vi "Get 1D Array String.vi"(5 "use temporary file? (F)":bool, 7 "data type of variable":string[](array[string]), 8 "error in":errorcluster, 10 "variable name":string, 11 "GOLPI ref. in":T1={"pipe handle"={"lv_proc.dll file path"=path "", "process instance handle"=[], "debug mode"=FALSE, "debug data"=[]}, "fast read timeout [ms]"=500, "fast read settle time [ms]"=10, "fast read to multiple [ms]"=1, "max elements per input line"=100, "slow read timeout [ms]"=5000, "stdin double format specifier"="%_16e", "max elements per stdout output column"=100, "console mode bitstream"=FALSE, "bitstream first read timeout [ms]"=1000, "bitstream read timeout [ms]"=50, "struct transfer possible"=FALSE, "matlab mode"=FALSE}) -> (0 "error out":errorcluster, 2 "value":string[](array[string]), 3 "GOLPI ref. out":T1={"pipe handle"={"lv_proc.dll file path"=path "", "process instance handle"=[], "debug mode"=FALSE, "debug data"=[]}, "fast read timeout [ms]"=500, "fast read settle time [ms]"=10, "fast read to multiple [ms]"=1, "max elements per input line"=100, "slow read timeout [ms]"=5000, "stdin double format specifier"="%_16e", "max elements per stdout output column"=100, "console mode bitstream"=FALSE, "bitstream first read timeout [ms]"=1000, "bitstream read timeout [ms]"=50, "struct transfer possible"=FALSE, "matlab mode"=FALSE})   [LabVIEW 2020, in "GOLPI library.lvlib"]
doc: "Part of polymorph Get Variable.vi"
uses:
  GOLPI library.lvlib
  GOLPI reference Type Def.ctl
  Pipe Handle.ctl
  Bitstream Data Type.ctl
  Custom Error Codes Enum Type Def.vi
  LV Process library.lvlib
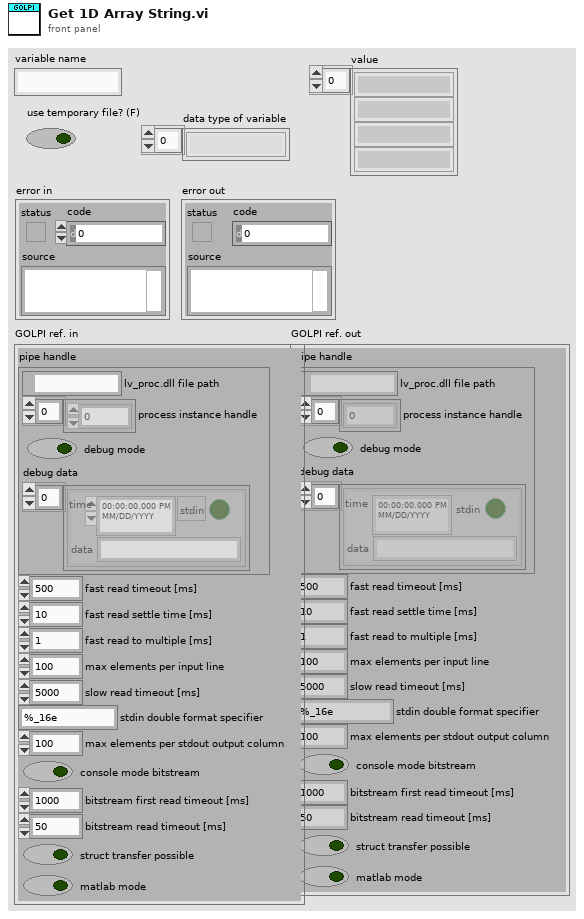
[diagram p1: front panel]
types:
  T1 = typedef "GOLPI library.lvlib/GOLPI reference Type Def.ctl" = cluster{"pipe handle":T2, "fast read timeout [ms]":u32, "fast read settle time [ms]":u32, "fast read to multiple [ms]":u32, "max elements per input line":u32, "slow read timeout [ms]":u32, "stdin double format specifier":string, "max elements per stdout output column":u32, "console mode bitstream":bool, "bitstream first read timeout [ms]":u32, "bitstream read timeout [ms]":u32, "struct transfer possible":bool, "matlab mode":bool}
  T2 = typedef "LV Process library.lvlib/Pipe Handle.ctl" = cluster{"lv_proc.dll file path":path, "process instance handle":u32[], "debug mode":bool, "debug data":cluster{"time":timestamp, "stdin":bool, "data":string}[]}
  T3 = typedef "GOLPI library.lvlib/Bitstream Data Type.ctl" = enum16{"dummy", "int", "uint", "float", "complex", "str", "real numeric"}
  T4 = typedef "GOLPI library.lvlib/Custom Error Codes Enum Type Def.vi" = enum16{"no error", "00 working directory PAR1 missing", "01 octave binary PAR1 missing", "02 octave report error PAR1", "03 empty output last cmd PAR1", "04 missing temporary file PAR1", "05 pwd PAR 1 not exist", "06 oct package not installed", "07 octave default binary missing", "10 var PAR1 not string, vect", "11 var PAR1 not num, scal, ~compl", "12 var PAR1 not num, scal, compl", "13 var PAR1 not num, vect, ~compl", "14 var PAR1 not num, vect, compl", "15 var PAR1 not num, mat, ~compl", "16 var PAR1 not num, mat, ~compl", "30 read timeout", "60 bitstream transport failed", "61 bitstream decode error PAR1", "62 bitstream cannot be set", "70 struct transfer not possible", "80 struct: cluster elem. PAR1 not implem.", "81 struct: structure field PAR1 not implem.", "82 struct: size mismatch of PAR1", "83 struct: type mismatch of PAR1", "98 internal error", "99 not finished", "90 Not supported in Matlab mode", "91 Matlab variable transfer error", "92 Matlab Script Error"}
  T5 = typedef "GOLPI library.lvlib/Bitstream Data.ctl" = cluster{"double":dbl[][], "cplx double":cdb[][], "int64":i64[][], "uint64":u64[][], "str":string[], "data type":T3}
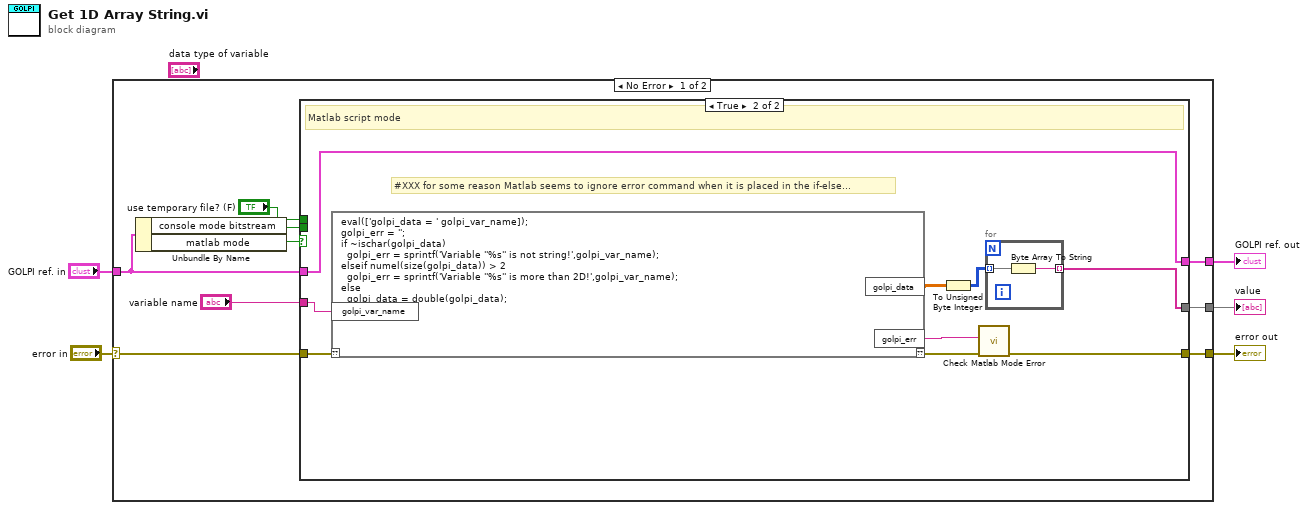
[diagram p0: block diagram]
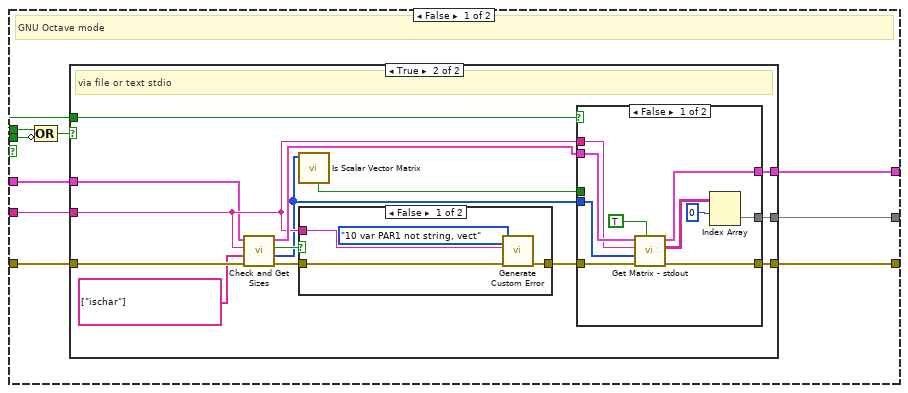
[diagram p2: hidden frame]
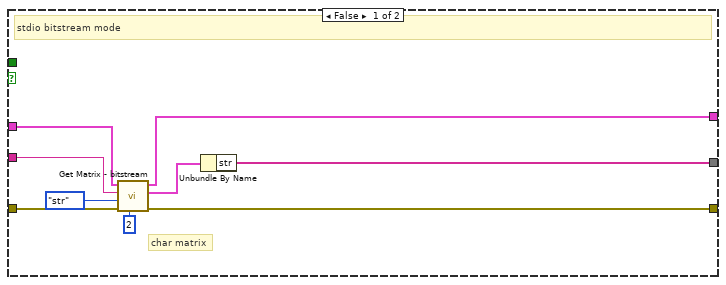
[diagram p3: hidden frame]
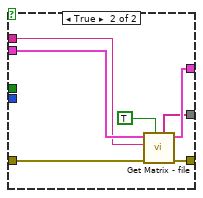
[diagram p4: hidden frame]
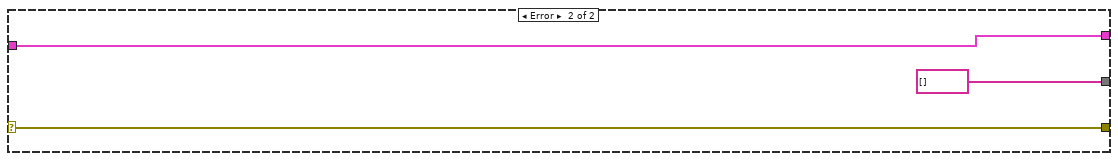
[diagram p6: hidden frame]
diagram:
  n1 = case shown="No Error" "error in" {
    selector: "error in" -> [w13 w82]
    tunnel: [w12 w82] -> w5
    tunnel: [w14 string[] [] ("vector")] -> w3
    tunnel: "GOLPI ref. in" -> [w9 w80]
    tunnel: [w10 w80] -> w1
    frame No Error {
      n2 = Unbundle By Name(w9) -> ("console mode bitstream"=w8:bool, "matlab mode"=w6:bool)
      n3 = case shown="True" w6 {
        tunnel: [w23 w72] -> w14
        tunnel: w13 -> [w22 w77]
        tunnel: [w21 w69] -> w12
        tunnel: "variable name" -> [w20 w76]
        tunnel: [w19 w75] -> w10
        tunnel: w9 -> [w18 w75]
        tunnel: w8 -> [w17 _]
        tunnel: "use temporary file? (F)" -> [w15 _]
        frame False {
          # "GNU Octave mode"
          n4 = Compound Arithmetic op=OR(w15, invert w17) -> (w16:bool)
          n5 = case shown="True" w16 {
            tunnel: [w25 w46] -> w23
            tunnel: w22 -> [w32 w44]
            tunnel: [w24 w39] -> w21
            tunnel: w20 -> [w29 w38]
            tunnel: w18 -> [w31 w37]
            tunnel: [w30 w36] -> w19
            tunnel: w15 -> [_ w33]
            frame False {
              # "char matrix"
              # "stdio bitstream mode"
              n6 = call "Get Matrix - bitstream.vi"("max dimensions (0: scalar)"=2, "error in (no error)"=w32, "data type"=Bitstream_Data_Type."str", "variable name"=w29, "GOLPI ref. in"=w31) -> ("error out"=w24:errorcluster, "data"=w26:T5, "GOLPI ref. out"=w30:T1)  [unwired: 4 in]
              n7 = Unbundle By Name(w26) -> ("str"=w25:string[])
            }
            frame True {
              # "via file or text stdio"
              n8 = call "Check and Get Sizes.vi"("error in (no error)"=w44, "test commands"=string[] ["ischar"], "variable name"=w38, "GOLPI ref. in"=w37) -> ("error out"=w43:errorcluster, "octave sizes"=w35:i32[], "all tests OK?"=w45:bool, "GOLPI ref. out"=w41:T1)  [unwired: 4 in]
              n9 = call "Is Scalar Vector Matrix.vi"("octave sizes"=w35) -> ("row vector?"=w34:bool)  [unwired: 5 in, 5 out]
              n10 = case shown="False" w45 {
                tunnel: w43 -> [w67 w68]
                tunnel: [w64 w68] -> w40
                tunnel: w38 -> [w65 _]
                frame False {
                  n11 = call "Generate Custom Error.vi"("error in"=w67, "PAR1"=w65, "GOLPI error"=Custom_Error_Codes_Enum_Type_Def.vi."10 var PAR1 not string, vect" ("Enum")) -> ("error out"=w64:errorcluster)  [unwired: 8 in]
                }
                frame True {
                }
              }
              n12 = case shown="False" w33 {
                tunnel: [w47 w58] -> w46
                tunnel: w41 -> [w56 w61]
                tunnel: w35 -> [w49 _]
                tunnel: w40 -> [w55 w63]
                tunnel: [w54 w62] -> w39
                tunnel: w38 -> [w48 w59]
                tunnel: [w53 w60] -> w36
                tunnel: w34 -> [_ _]
                frame False {
                  n13 = call "Get Matrix - stdout.vi"("is string?"=TRUE ("is string"), "error in (no error)"=w55, "octave sizes"=w49, "variable name"=w48, "GOLPI ref. in"=w56) -> ("error out"=w54:errorcluster, "array"=w50:string[][], "GOLPI ref. out"=w53:T1)  [unwired: 4 in]
                  n14 = Index Array(array=w50, index (row)=0) -> (element=w47:string[])  [unwired: 1 in]
                }
                frame True {
                  n15 = call "Get Matrix - file.vi"("is string?"=TRUE ("is string"), "error in (no error)"=w63, "variable name"=w59, "GOLPI ref. in"=w61) -> ("error out"=w62:errorcluster, "GOLPI ref. out"=w60:T1, "string array"=w58:string[])  [unwired: 3 in, 2 out]
                }
              }
            }
          }
        }
        frame True {
          # "#XXX for some reason Matlab seems to ignore error command when it is placed in the if-else..."
          # "Matlab script mode"
          n16 = script code="eval(['golpi_data = ' golpi_var_name]);\ngolpi_err = '';\nif ~ischar(golpi_data)\n  golpi_err = sprintf('Variable ''%s'' is not string!',golpi_var_name);  \nelseif numel(size(golpi_data)) > 2\n  golpi_err = sprintf('Variable ''%s'' is more than 2D!',golpi_var_name);  \nelse\n  golpi_data = double(golpi_data);\nend"("??"=w77, "golpi_var_name"=w76) -> ("??"=w71:errorcluster, "golpi_data"=w74:dbl[][], "golpi_err"=w70:string)
          n17 = To Unsigned Byte Integer(number=w74) -> (unsigned 8bit integer=w73:u8[][])
          n18 = call "Check Matlab Mode Error.vi"("error in"=w71, "custom error string (empty)"=w70) -> ("error out"=w69:errorcluster)  [unwired: 9 in]
          n19 = for {
            tunnel: w73 -> [w79] mode=indexing
            tunnel: [w78] -> w72 mode=indexing
            n20 = Byte Array To String(unsigned byte array=w79) -> (string=w78:string)
          }
        }
      }
    }
    frame Error {
    }
  }
  "value" <- w3
  "error out" <- w5
  "GOLPI ref. out" <- w1
